vi "DB Tools Delete Data.vi"(7 "condition":string, 8 "error in (no error)":errorcluster, 10 "table":string, 11 "connection reference":T1) -> (0 "error out":errorcluster, 3 "connection reference out":T1)   [LabVIEW 2020, in "NI_Database_API.lvlib"]
doc: "Deletes data from a database identified by <B>connection reference</B>."
uses:
  <vilib>/addons/database/NI_Database_API.lvlib
  <vilib>/addons/database/Connection.llb/Conn ObjectReference.ctl
  <vilib>/addons/database/Connection.llb/Conn Execute.vi
  <vilib>/addons/database/Recordset.llb/Rec Destroy - Connection.vi
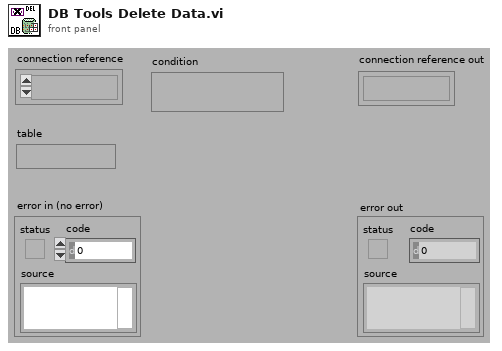
[diagram p1: front panel]
types:
  T1 = typedef "NI_Database_API.lvlib/Conn ObjectReference.ctl" = refnum<k1>
  T2 = typedef "NI_Database_API.lvlib/Rec ObjectReference.ctl" = refnum<k1>
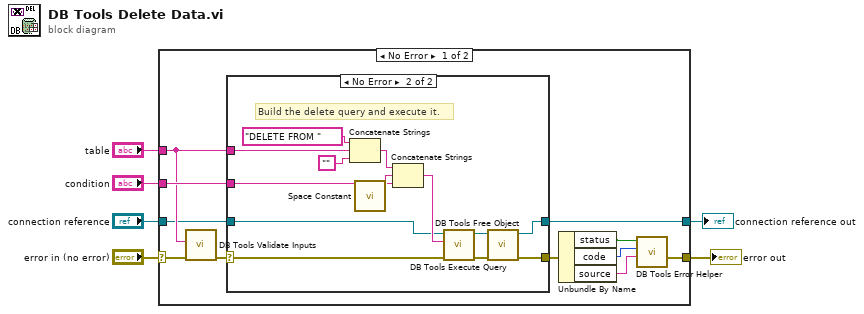
[diagram p0: block diagram]
diagram:
  n1 = case shown="No Error" "error in (no error)" {
    selector: "error in (no error)" -> [w7 w34]
    tunnel: [w17 w33] -> w6
    tunnel: [w12 w34] -> w5
    tunnel: "condition" -> [w11 _]
    tunnel: "table" -> [w10 _]
    tunnel: "connection reference" -> [w9 w33]
    frame No Error {
      n2 = call <vilib>:"DB Tools Validate Inputs.vi"("error in (no error)"=w7, "table"=w10) -> ("error out"=w8:errorcluster)  [unwired: 3 in, 2 out]
      n3 = case shown="No Error" w8 {
        selector: w8 -> [w19 w20]
        tunnel: [w18 w32] -> w17
        tunnel: [w19 w31] -> w13
        tunnel: w11 -> [_ w29]
        tunnel: w10 -> [_ w26]
        tunnel: w9 -> [w18 w23]
        frame Error {
          # "No table is specified; output error."
        }
        frame No Error {
          # "Build the delete query and execute it."
          n4 = Concatenate Strings("DELETE FROM " ("Substring"), w26, "") -> (w25:string)
          n5 = call <vilib>:"Space Constant.vi"() -> ("String"=w30:string)
          n6 = Concatenate Strings(w25, w30, w29) -> (w24:string)
          n7 = call-poly <vilib>:"DB Tools Execute Query.vi"("error in (no error)"=w20, "SQL query"=w24, "connection reference"=w23) -> ("error out"=w21:errorcluster, "recordset reference"=w22:T2)  [unwired: 5 in]
          n8 = call-poly <vilib>:"DB Tools Free Object.vi"("error in (no error)"=w21, "recordset reference"=w22) -> ("error out"=w31:errorcluster, "connection reference"=w32:T1)  [unwired: 8 in]
        }
      }
      n9 = Unbundle By Name(w13) -> ("status"=w16:bool, "code"=w15:i32, "source"=w14:string)
      n10 = call <vilib>:"DB Tools Error Helper.vi"("source"=w14, "code"=w15, "status"=w16) -> ("error out"=w12:errorcluster)  [unwired: 8 in]
    }
    frame Error {
    }
  }
  "error out" <- w5
  "connection reference out" <- w6
